vi "main.vi"() -> ()   [LabVIEW 2021]
uses:
  Operation.ctl
panel:
  out "PrevResult":string
  out "Result":string
  out "LastOperation":T1
  in  "Button C":bool
  in  "Stop":bool
  in  "Button Compute":bool
  in  "Button Dot":bool
  in  "Button 0":bool
  in  "Button Sign":bool
  in  "Button Plus":bool
  in  "Button Minus":bool
  in  "Button Mult":bool
  in  "Button Div":bool
  in  "Button 9":bool
  in  "Button 8":bool
  in  "Button 7":bool
  in  "Button 6":bool
  in  "Button 5":bool
  in  "Button 4":bool
  in  "Button 3":bool
  in  "Button 2":bool
  in  "Button 1":bool
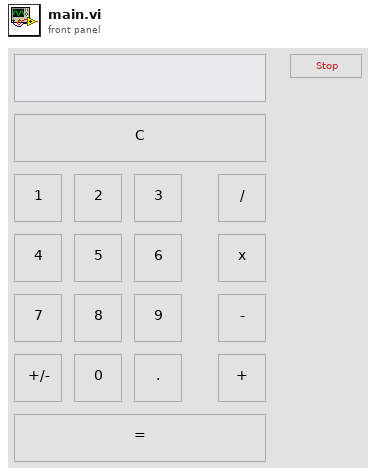
[diagram p1: front panel]
types:
  T1 = typedef "Operation.ctl" = enum16{"Plus", "Minus", "Multiply", "Divide"}
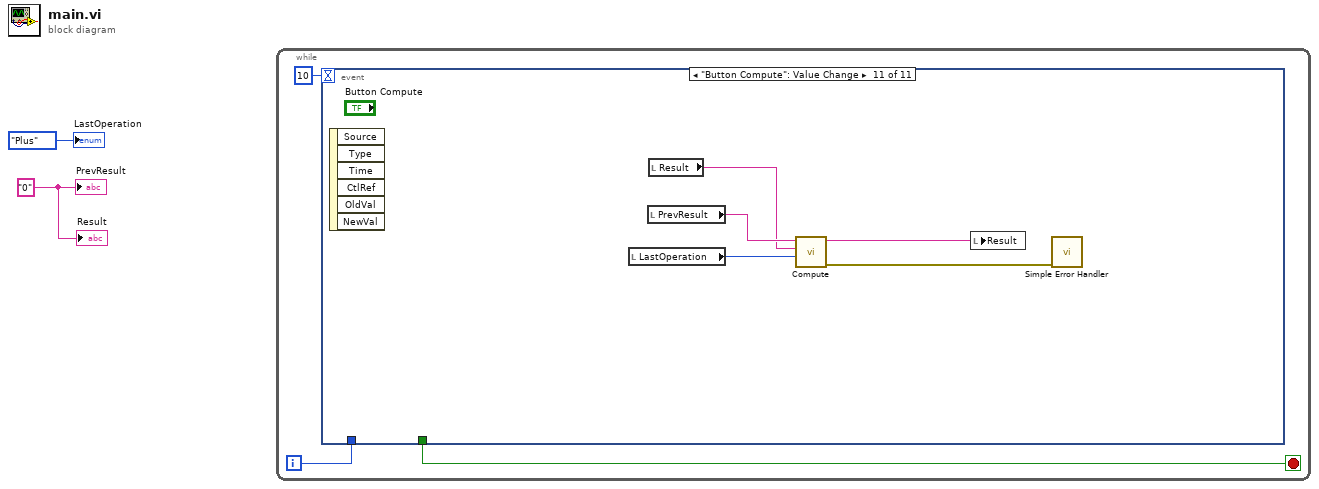
[diagram p0: block diagram]
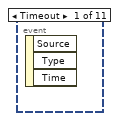
[diagram p2: hidden frame]
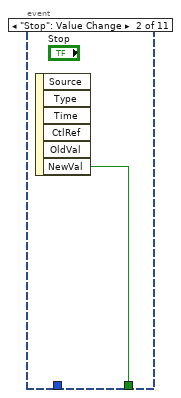
[diagram p3: hidden frame]
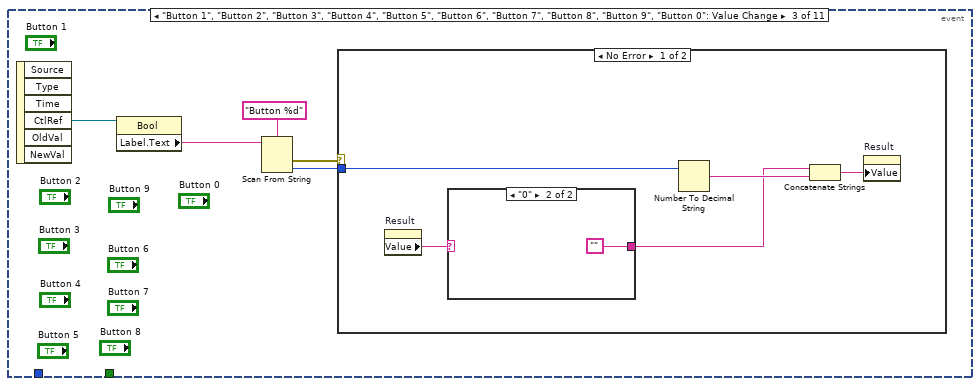
[diagram p4: hidden frame]
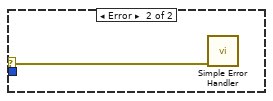
[diagram p6: hidden frame]
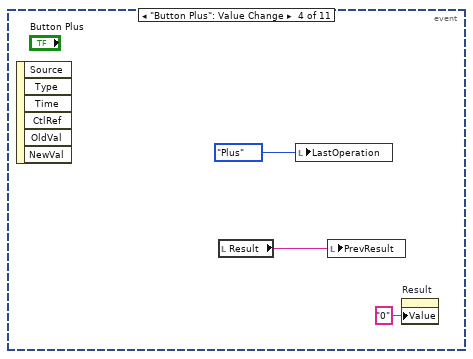
[diagram p7: hidden frame]
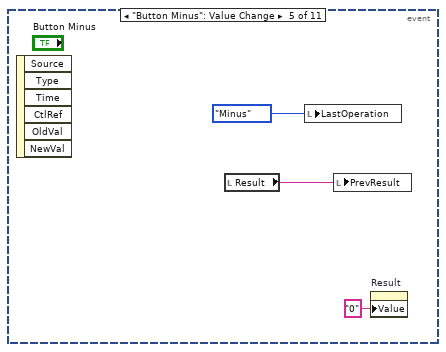
[diagram p8: hidden frame]
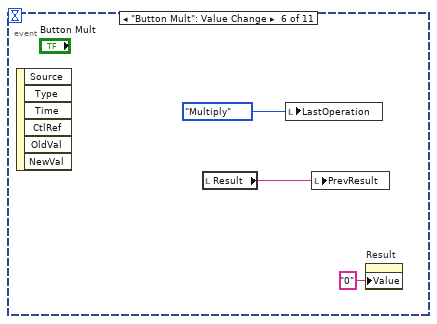
[diagram p9: hidden frame]
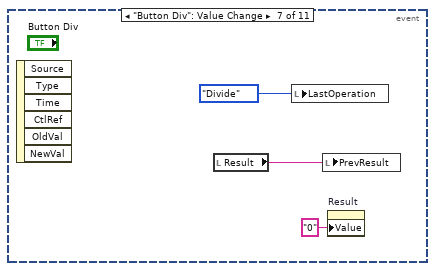
[diagram p10: hidden frame]
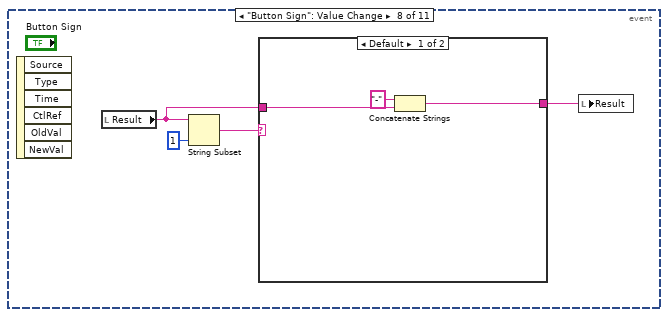
[diagram p11: hidden frame]
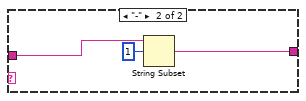
[diagram p12: hidden frame]
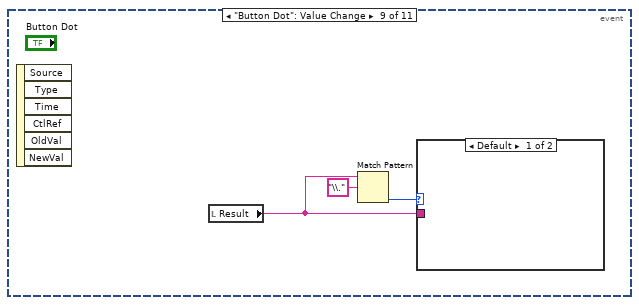
[diagram p13: hidden frame]
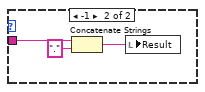
[diagram p14: hidden frame]
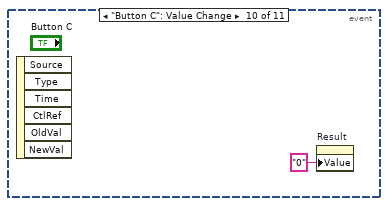
[diagram p15: hidden frame]
diagram:
  w1 = "0" ("PrevResult")
  n1 = while {
    i -> [w3]
    stop <- w5 stop-if-true
    n2 = event shown="[10] \"Button Compute\": Value Change" {
      selector: _ -> [_ _ _ _ _ _ _ _ _ _ _]
      dyn-events: _ -> [_ _ _ _ _ _ _ _ _ _ _]
      timeout: 10 -> [_ _ _ _ _ _ _ _ _ _ _]
      tunnel: [_ w6 _ _ _ _ _ _ _ _ _] -> w5
      tunnel: w3 -> [_ _ _ _ _ _ _ _ _ _ _]
      event Timeout {
        n3 = event-data() -> ()  [unwired: 1 in, 3 out]
      }
      event "Stop": Value Change {
        n4 = event-data() -> ("NewVal"=w6:bool)  [unwired: 1 in, 5 out]
      }
      event "Button 1", "Button 2", "Button 3", "Button 4", "Button 5", "Button 6", "Button 7", "Button 8", "Button 9", "Button 0": Value Change {
        n5 = event-data() -> ("CtlRef"=w10:refnum<vi>)  [unwired: 1 in, 5 out]
        n6 = property class="Bool"(reference=w10) -> ("Label.Text"=w8:string)  [unwired: 1 in, 2 out]
        n7 = Scan From String(format string="Button %d", input string=w8) -> (error out=w7:errorcluster, output 1=w9:i32)  [unwired: 3 in, 2 out]
        n8 = case shown="No Error" w7 {
          selector: w7 -> [_ w19]
          tunnel: w9 -> [w14 _]
          frame No Error {
            n9 = property on="Result" class="Str"() -> ("Value"=w13:string)  [unwired: 2 in, 2 out]
            n10 = case shown="\"0\"" w13 {
              selector: w13 -> [w17 _]
              tunnel: [w17 ""] -> w12
              frame Default {
              }
              frame "0" {
              }
            }
            n11 = Number To Decimal String(number=w14) -> (decimal integer string=w16:string)  [unwired: 1 in]
            n12 = Concatenate Strings(w12, w16) -> (w15:string)
            n13 = property on="Result" class="Str"("Value"=w15) -> ()  [unwired: 2 in, 2 out]
          }
          frame Error {
            n14 = call <vilib>:"Simple Error Handler.vi"("error in (no error)"=w19) -> ()  [unwired: 4 in, 5 out]
          }
        }
      }
      event "Button Plus": Value Change {
        n15 = event-data() -> ()  [unwired: 1 in, 6 out]
        n16 = local read "Result"() -> (w21:string)
        n17 = local write "LastOperation"(Operation."Plus" ("LastOperation")) -> ()
        n18 = local write "PrevResult"(w21) -> ()
        n19 = property on="Result" class="Str"("Value"="0" ("Result")) -> ()  [unwired: 2 in, 2 out]
      }
      event "Button Minus": Value Change {
        n20 = event-data() -> ()  [unwired: 1 in, 6 out]
        n21 = local read "Result"() -> (w24:string)
        n22 = local write "LastOperation"(Operation."Minus" ("LastOperation")) -> ()
        n23 = local write "PrevResult"(w24) -> ()
        n24 = property on="Result" class="Str"("Value"="0" ("Result")) -> ()  [unwired: 2 in, 2 out]
      }
      event "Button Mult": Value Change {
        n25 = event-data() -> ()  [unwired: 1 in, 6 out]
        n26 = local read "Result"() -> (w27:string)
        n27 = local write "LastOperation"(Operation."Multiply" ("LastOperation")) -> ()
        n28 = local write "PrevResult"(w27) -> ()
        n29 = property on="Result" class="Str"("Value"="0" ("Result")) -> ()  [unwired: 2 in, 2 out]
      }
      event "Button Div": Value Change {
        n30 = event-data() -> ()  [unwired: 1 in, 6 out]
        n31 = local read "Result"() -> (w30:string)
        n32 = local write "LastOperation"(Operation."Divide" ("LastOperation")) -> ()
        n33 = local write "PrevResult"(w30) -> ()
        n34 = property on="Result" class="Str"("Value"="0" ("Result")) -> ()  [unwired: 2 in, 2 out]
      }
      event "Button Sign": Value Change {
        n35 = event-data() -> ()  [unwired: 1 in, 6 out]
        n36 = local read "Result"() -> (w32:string)
        n37 = String Subset(string=w32, length (rest)=1 ("length (rest)")) -> (substring=w34:string)  [unwired: 1 in]
        n38 = case shown="Default" w34 {
          tunnel: [w36 w40] -> w33
          tunnel: w32 -> [w38 w39]
          frame Default {
            n39 = Concatenate Strings("-" ("string"), w38) -> (w36:string)
          }
          frame "-" {
            n40 = String Subset(string=w39, offset (0)=1) -> (substring=w40:string)  [unwired: 1 in]
          }
        }
        n41 = local write "Result"(w33) -> ()
      }
      event "Button Dot": Value Change {
        n42 = event-data() -> ()  [unwired: 1 in, 6 out]
        n43 = local read "Result"() -> (w44:string)
        n44 = Match Pattern(string=w44, regular expression="\\.") -> (offset past match=w42:i32)  [unwired: 1 in, 3 out]
        n45 = case shown="Default" w42 {
          tunnel: w44 -> [_ w45]
          frame Default {
          }
          frame -1 {
            n46 = Concatenate Strings(w45, "." ("string")) -> (w46:string)
            n47 = local write "Result"(w46) -> ()
          }
        }
      }
      event "Button C": Value Change {
        n48 = event-data() -> ()  [unwired: 1 in, 6 out]
        n49 = property on="Result" class="Str"("Value"="0" ("Result")) -> ()  [unwired: 2 in, 2 out]
      }
      event "Button Compute": Value Change {
        n50 = event-data() -> ()  [unwired: 1 in, 6 out]
        n51 = local read "LastOperation"() -> (w53:T1)
        n52 = local read "PrevResult"() -> (w50:string)
        n53 = local read "Result"() -> (w49:string)
        n54 = call "Compute.vi"("Operation"=w53, "Operand2"=w49, "Operand1"=w50) -> ("error out"=w51:errorcluster, "Result"=w52:string)  [unwired: 7 in]
        n55 = local write "Result"(w52) -> ()
        n56 = call <vilib>:"Simple Error Handler.vi"("error in (no error)"=w51) -> ()  [unwired: 4 in, 5 out]
      }
    }
  }
  "LastOperation" <- Operation."Plus" ("Operation")
  "PrevResult" <- w1
  "Result" <- w1
